vi "Log Result.vi"(8 "error in (no error)":errorcluster, 10 "Result":refnum<class "Acquired Result.lvclass">, 11 "File in":refnum<class "File.lvclass">) -> (0 "error out":errorcluster, 3 "File out":refnum<class "File.lvclass">)   [LabVIEW 2016, in "File.lvclass"]
uses:
  File.lvclass
  Instruments/Results/Acquired Result/Acquired Result.lvclass
  File.lvclass/File.ctl
  Read tdms stream.vi
  Read Timestamp data points.vi
  Write tdms stream.vi
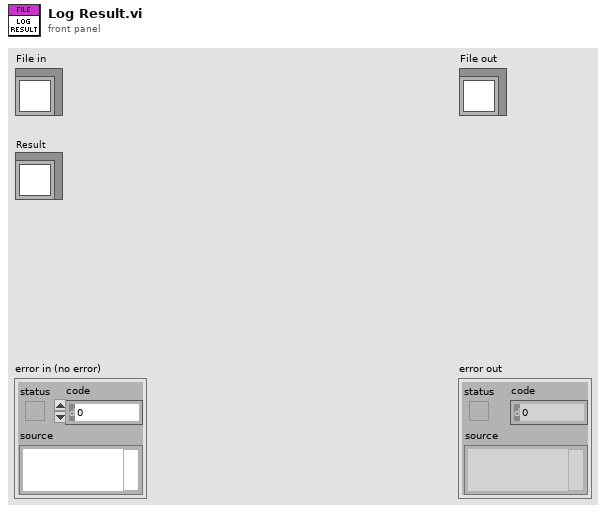
[diagram p1: front panel]
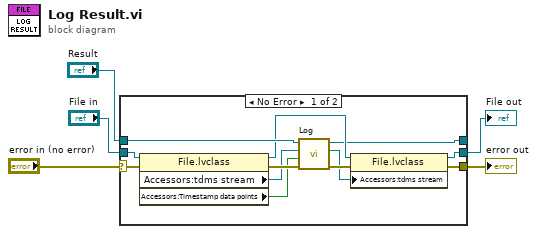
[diagram p0: block diagram]
diagram:
  n1 = case shown="No Error" "error in (no error)" {
    selector: "error in (no error)" -> [w13 w20]
    tunnel: [w12 w20] -> w2
    tunnel: [w8 w19] -> w3
    tunnel: "File in" -> [w9 w19]
    tunnel: "Result" -> [w11 w18]
    tunnel: [w7 w18] -> _
    frame No Error {
      n2 = property class="File.lvclass"(reference=w9, error in=w13) -> (reference out=w10:refnum<class "File.lvclass">, error out=w16:errorcluster, "Accessors:tdms stream"=w14:refnum<k34>, "Accessors:Timestamp data points"=w6:bool)
      n3 = call-dynamic "Log.vi"("error in (no error)"=w16, "Timestamp data points"=w6, "tdms file"=w14, "Acquired Result in"=w11) -> ("error out"=w17:errorcluster, "tdms file out"=w15:refnum<k34>, "Acquired Result out"=w7:refnum<class "Acquired Result.lvclass">)  [unwired: 5 in]
      n4 = property class="File.lvclass"(reference=w10, error in=w17, "Accessors:tdms stream"=w15) -> (reference out=w8:refnum<class "File.lvclass">, error out=w12:errorcluster)
    }
    frame Error {
    }
  }
  "error out" <- w2
  "File out" <- w3
